vi "Seconds Till Stop.vi"(10 "i":dbl, 11 "Time":dbl) -> (3 "x >= y?":bool)   [LabVIEW 2015]
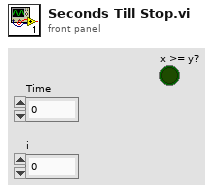
[diagram p1: front panel]
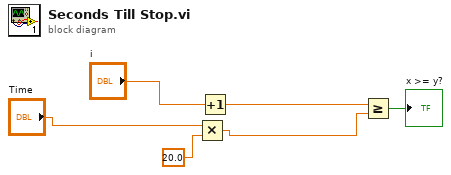
[diagram p0: block diagram]
diagram:
  n1 = Multiply(x="Time", y=20.0) -> (x*y=w3:dbl)
  n2 = Increment(x="i") -> (x+1=w1:dbl)
  n3 = Greater Or Equal?(x=w1, y=w3) -> (x >= y?=→"x >= y?":bool)
